vi "Modified Write To SGL File.vi"(6 "append to file? (new file:F)":bool, 7 "Interactive":bool=TRUE, 8 "error in (no error)":errorcluster, 9 "1D array":sgl[](array[numeric]) format="%.2f", 10 "2D array":sgl[][](array[numeric]) format="%.3f", 11 "file path (dialog if empty)":path) -> (0 "error out":errorcluster, 5 "new file path (Not A Path if cancelled)":path)   [LabVIEW 2015]
doc: "Writes a 2D or 1D array of single-precision numbers (SGL) to a new byte stream file or appends the data to an existing file. The VI opens or creates the file beforehand and closes it afterwards. You can use this VI to write scaled data from data acquisition VIs.\n\nfile path is the path name of the file. If file path is empty (default value) or is Not A Path, the VI displays a File dialog box from which you can select a file. Error 43 occurs if the user cancels the dialog. \n\n2D data contains the single-precision numbers the VI writes to the file if 1D data is not wired or empty.\n\n1D data contains the single-precision numbers the VI writes to the file if this input is not empty.\n\nappend to file? Set to TRUE if you want to append the data to a existing file; you can also set it TRUE to write to a new file. Set to FALSE (default value) if you want to write the data to a new file or to replace an existing file.\n\nnew file path is the path of the file to which the VI wrote data. You can use this output to determine the path of a file that you open using dialog. new file path returns Not A Path if the user selects Cancel from the dialog box."
panel:
  in  "prompt":string="Choose file to write."
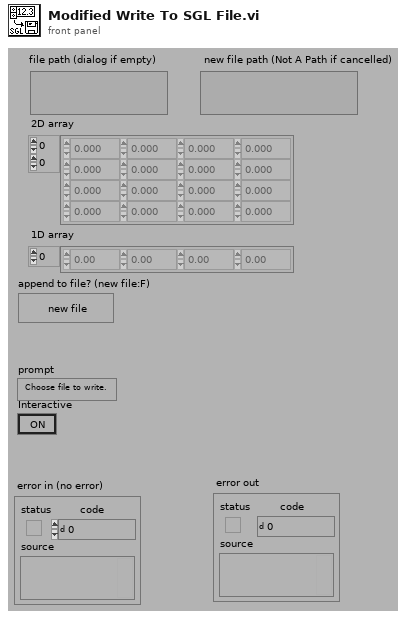
[diagram p1: front panel]
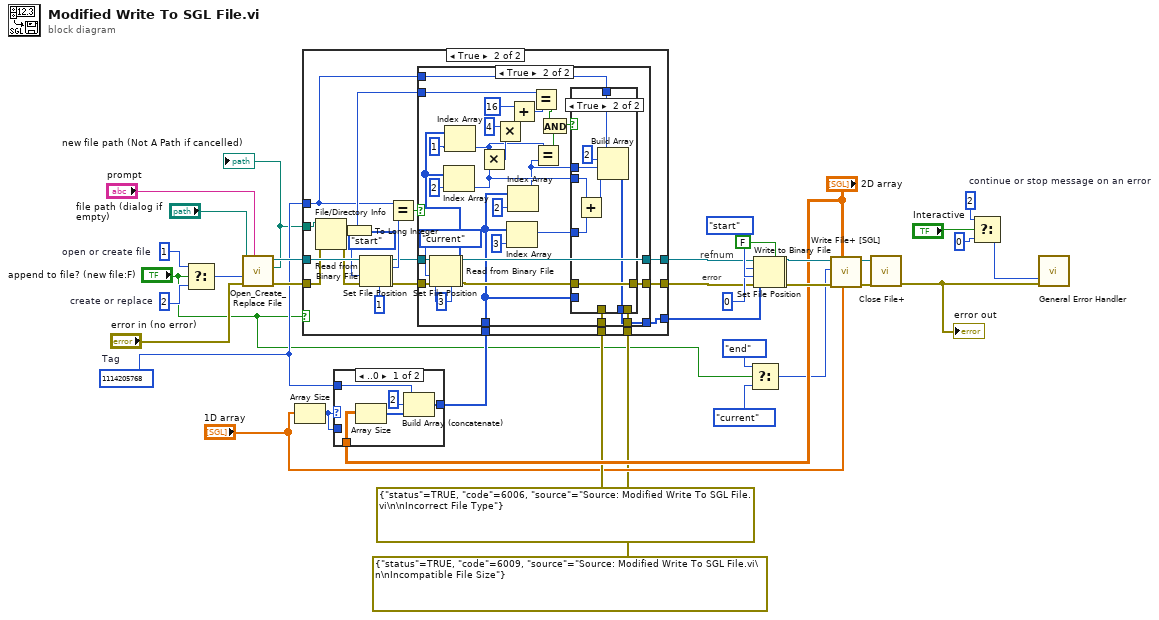
[diagram p0: block diagram]
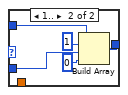
[diagram p5: hidden frame]
diagram:
  w17 = 1114205768  # Tag
  w32 = i16 2  # create or replace
  w29 = 2  # continue or stop message on an error
  w33 = i16 1  # open or create file
  # "error"
  # "refnum"
  n1 = Select(t=w33, s="append to file? (new file:F)", f=w32) -> (s? t:f=w34:i16)
  n2 = call <vilib>:"Open_Create_Replace File.vi"("prompt"="prompt", "error in (no error)"="error in (no error)", "function (open:0)"=w34, "file path"="file path (dialog if empty)") -> ("error out"=w19:errorcluster, "new file path"=w13:path, "refnum"=w18:refnum<file>)  [unwired: 4 in, 1 out]
  "new file path (Not A Path if cancelled)" <- w13
  n3 = Array Size(array="1D array") -> (size(s)=w9:i32)
  n4 = case shown="..0" w9 {
    tunnel: "2D array" -> [w42 _]
    tunnel: [w39 w46] -> w12
    tunnel: w17 -> [w38 w45]
    tunnel: w9 -> [_ w43]
    frame ..0 {
      n5 = Array Size(array=w42) -> (size(s)=w41:i32[])
      n6 = Build Array (concatenate)(w38, 2 ("Input Element"), w41) -> (w39:i32[])
    }
    frame 1.. {
      n7 = Build Array(w45, 1 ("Input Element"), w43, 0 ("Input Element")) -> (w46:i32[])
    }
  }
  n8 = case shown="True" "append to file? (new file:F)" {
    tunnel: w19 -> [w49 w60]
    tunnel: w18 -> [w50 w71]
    tunnel: w17 -> [_ w55]
    tunnel: [w49 w66] -> w16
    tunnel: errorcluster {"status"=TRUE, "code"=6006, "source"="Source: Modified Write To SGL File.vi\n\nIncorrect File Type"} ("error out") -> [_ w65]
    tunnel: [w50 w64] -> w14
    tunnel: w13 -> [_ w61]
    tunnel: w12 -> [w48 w57]
    tunnel: [w48 w56] -> w11
    tunnel: errorcluster {"status"=TRUE, "code"=6009, "source"="Source: Modified Write To SGL File.vi\n\nIncompatible File Size"} ("error out") -> [_ w54]
    frame False {
    }
    frame True {
      n9 = File/Directory Info(path=w61, error in=w60) -> (size=w53:i64, error out=w59:errorcluster)  [unwired: 5 out]
      n10 = To Long Integer(number=w53) -> (32bit integer=w58:i32)
      n11 = Set File Position(refnum=w71, from (0:start)=enum16{"start", "end", "current"}."start" ("pos mode (0:2)"), error in=w59) -> (refnum out=w52:refnum<file>, error out=w51:errorcluster)  [unwired: 1 in]
      n12 = Read from Binary File(5:1 ("count"), 8:w51, 11:w52) -> (0:w62:errorcluster, 2:w69:i32, 3:w63:refnum<file>)  [unwired: 3 in, 1 out]
      n13 = Equal?(x=w55, y=w69) -> (x = y?=w67:bool)
      n14 = case shown="True" w67 {
        tunnel: [w74 w87] -> w66
        tunnel: w65 -> [w74 w86]
        tunnel: [w73 w85] -> w64
        tunnel: w63 -> [w73 w105]
        tunnel: w62 -> [_ w102]
        tunnel: w58 -> [_ w95]
        tunnel: w57 -> [w72 w78]
        tunnel: [w72 w79] -> w56
        tunnel: w55 -> [_ w81]
        tunnel: w54 -> [_ w77]
        frame False {
        }
        frame True {
          w103 = 3 ("count")
          n15 = Set File Position(refnum=w105, from (0:start)=enum16{"start", "end", "current"}."current" ("pos mode (0:2)"), error in=w102) -> (refnum out=w76:refnum<file>, error out=w75:errorcluster)  [unwired: 1 in]
          n16 = Read from Binary File(5:w103, 8:w75, 10:w103, 11:w76) -> (0:w88:errorcluster, 2:w106:i32[], 3:w85:refnum<file>)  [unwired: 2 in, 1 out]
          n17 = Index Array(array=w106, index=2 ("Index")) -> (element=w84:i32)
          n18 = Index Array(array=w106, index=1 ("Index")) -> (element=w93:i32)
          n19 = Multiply(x=w93, y=w84) -> (x*y=w99:i32)
          n20 = Multiply(x=4, y=w99) -> (x*y=w97:i32)
          n21 = Index Array(array=w78, index=3 ("Index")) -> (element=w82:i32)
          n22 = Index Array(array=w78, index=2 ("Index")) -> (element=w80:i32)
          n23 = Add(x=16, y=w97) -> (x+y=w94:i32)
          n24 = Equal?(x=w95, y=w94) -> (x = y?=w91:bool)
          n25 = Equal?(x=w93, y=w80) -> (x = y?=w90:bool)
          n26 = And(x=w91, y=w90) -> (x .and. y?=w89:bool)
          n27 = case shown="True" w89 {
            tunnel: w88 -> [_ w116]
            tunnel: [w107 w116] -> w87
            tunnel: w86 -> [_ _]
            tunnel: w84 -> [_ w115]
            tunnel: w82 -> [_ w114]
            tunnel: w81 -> [_ w112]
            tunnel: w80 -> [_ w110]
            tunnel: [w108 w109] -> w79
            tunnel: w78 -> [w108 _]
            tunnel: w77 -> [w107 _]
            frame False {
            }
            frame True {
              n28 = Add(x=w115, y=w114) -> (x+y=w111:i32)
              n29 = Build Array(w112, 2 ("Input Element"), w110, w111) -> (w109:i32[])
            }
          }
        }
      }
    }
  }
  n30 = Select(t=enum16{"start", "end", "current"}."end" ("pos mode (rel. to end:1)"), s="append to file? (new file:F)", f=enum16{"start", "end", "current"}."current" ("pos mode (rel. to end:1)")) -> (s? t:f=w4:enum16{"start", "end", "current"})
  n31 = Set File Position(offset (in bytes) (0)=0 ("pos offset (0)"), refnum=w14, from (0:start)=enum16{"start", "end", "current"}."start" ("pos mode (0:2)"), error in=w16) -> (refnum out=w3:refnum<file>, error out=w2:errorcluster)
  n32 = Write to Binary File(file (use dialog)=w3, data=w11, error in=w2, 5:FALSE ("prepend array or string size? (T)")) -> (refnum out=w25:refnum<file>, error out=w26:errorcluster)  [unwired: 2 in, 1 out]
  n33 = call <vilib>:"Write File+ [SGL].vi"("1D array"="1D array", "2D array"="2D array", "error in (no error)"=w26, "pos mode (rel. to end:1)"=w4, "refnum"=w25) -> ("error out"=w36:errorcluster, "dup refnum"=w35:refnum<file>)  [unwired: 4 in, 1 out]
  n34 = call <vilib>:"Close File+.vi"("error in (no error)"=w36, "refnum"=w35) -> ("error out"=w20:errorcluster)  [unwired: 3 in, 2 out]
  "error out" <- w20
  n35 = Select(t=w29, s="Interactive", f=0) -> (s? t:f=w27:i32)
  n36 = call <vilib>:"General Error Handler.vi"("type of dialog (OK msg:1)"=w27, "error in (no error)"=w20) -> ()  [unwired: 9 in, 5 out]
